vi "ElmoVelOutScale.vi"(1 "vel (rad/s)":dbl) -> (0 "vel (tick/s)":dbl)   [LabVIEW 2018]
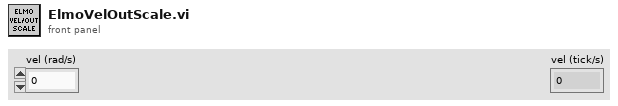
[diagram p1: front panel]
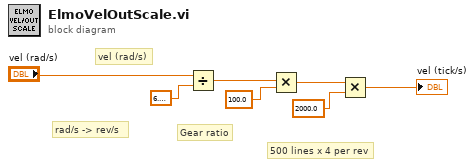
[diagram p0: block diagram]
diagram:
  # "rad/s -> rev/s"
  # "vel (rad/s)"
  # "500 lines x 4 per rev"
  # "Gear ratio"
  n1 = Divide(x="vel (rad/s)", y=6.283185307179586) -> (x/y=w3:dbl)
  n2 = Multiply(x=w3, y=100.0) -> (x*y=w6:dbl)
  n3 = Multiply(x=w6, y=2000.0) -> (x*y=→"vel (tick/s)":dbl)
